vi "PID SP Limiter.vi"(7 "SpLim_State":T2, 8 "REG param":T3={"proportional gain (Kc)"=1.0, "integral time (Ti, s)"=10.0, "derivative time (Td, s)"=1.0, "output high"=100.0, "output high start"=40.0, "output high stop"=40.0, "alr value"=0.0, "output low"=0.0, "output rate (EGU/s)"=5.0, "setpoint max"=100.0, "setpoint rate (EGU/min)"=10.0, "stop rate (EGU/min)"=5.0} {"setpoint max" format="%.2f"; "stop rate (EGU/min)" min=0.001 format="%.2f"; "setpoint rate (EGU/min)" min=0.001 format="%.2f"; "output high stop" format="%.2f"; "output high start" format="%.2f"; "output rate (EGU/s)" min=0.001 format="%.2f"; "output low" format="%.2f"; "alr value" format="%.2f"; "output high" format="%.2f"; "derivative time (Td, s)" format="%.3f"; "integral time (Ti, s)" format="%.3f"; "proportional gain (Kc)" format="%.3f"}, 10 "PV":dbl, 11 "SP":dbl) -> (0 "PID param":T1 {"dt (s)" format="%.3f"; "output rate (EGU/s)" format="%.2f"; "output low" format="%.2f"; "alr value" format="%.2f"; "output high" format="%.2f"; "derivative time (Td, s)" format="%.3f"; "integral time (Ti, s)" format="%.3f"; "proportional gain (Kc)" format="%.3f"}, 1 "End":bool, 2 "T":u32, 3 "output":dbl format="%.2f")   [LabVIEW 2019, in "control.lvlib"]
uses:
  control.lvlib
  ctl/control param.ctl
  ctl/SpLim_State.ctl
  ctl/PID param.ctl
  PID Timing Estimation.vi
panel:
  # "PID gains"
  # "output param"
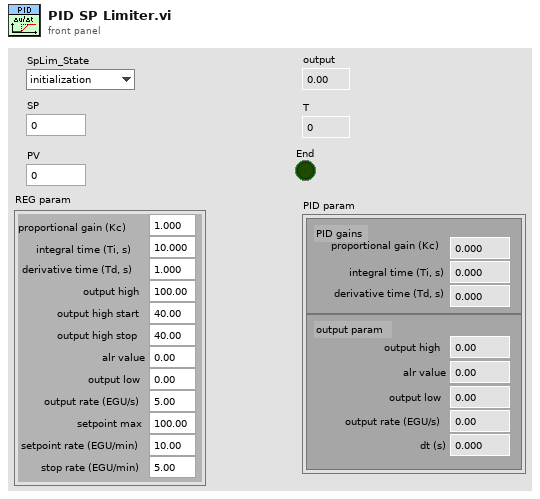
[diagram p1: front panel]
types:
  T1 = typedef "control.lvlib/PID param.ctl" = cluster{"proportional gain (Kc)":dbl, "integral time (Ti, s)":dbl, "derivative time (Td, s)":dbl, "output high":dbl, "alr value":dbl, "output low":dbl, "output rate (EGU/s)":dbl, "dt (s)":dbl}
  T2 = typedef "control.lvlib/SpLim_State.ctl" = enum8{"initialization", "stop", "decrease", "increase"}
  T3 = typedef "control.lvlib/control param.ctl" = cluster{"proportional gain (Kc)":dbl, "integral time (Ti, s)":dbl, "derivative time (Td, s)":dbl, "output high":dbl, "output high start":dbl, "output high stop":dbl, "alr value":dbl, "output low":dbl, "output rate (EGU/s)":dbl, "setpoint max":dbl, "setpoint rate (EGU/min)":dbl, "stop rate (EGU/min)":dbl}
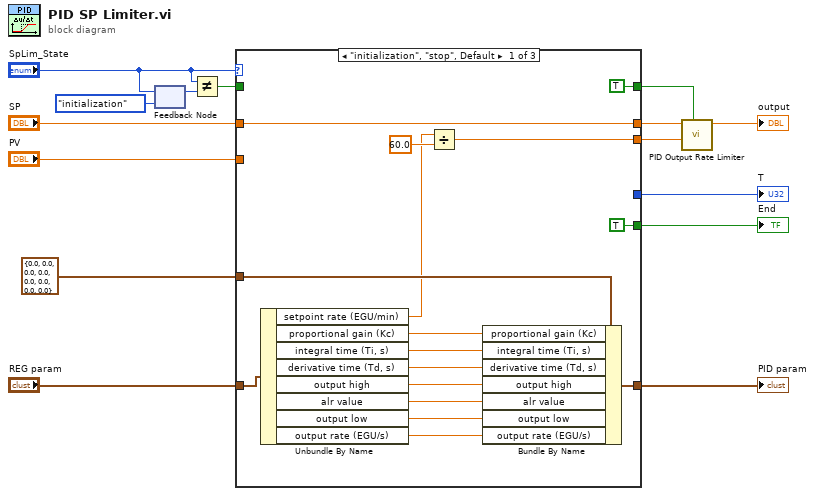
[diagram p0: block diagram]
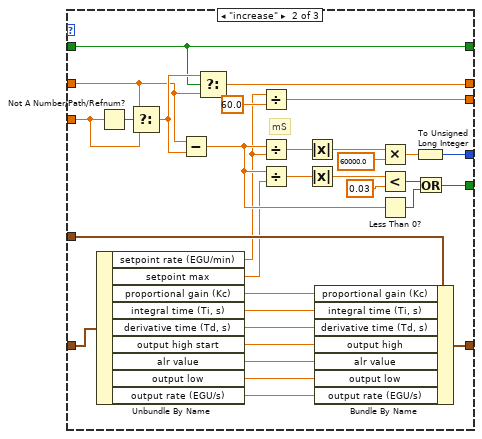
[diagram p2: hidden frame]
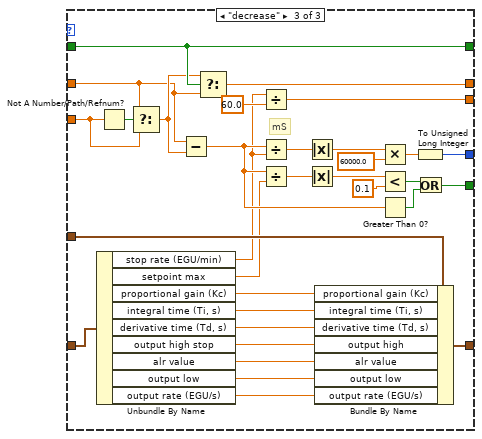
[diagram p3: hidden frame]
diagram:
  n1 = feedback #1(SpLim_State."initialization" ("SpLim_State")) -> (w7:T2)
  n2 = feedback-in #1("SpLim_State") -> ()
  n3 = Not Equal?(x="SpLim_State", y=w7) -> (x != y?=w8:bool)
  n4 = case shown="\"initialization\", \"stop\", Default" "SpLim_State" {
    tunnel: "SP" -> [w31 w37 w67]
    tunnel: "PV" -> [_ w62 w94]
    tunnel: [w31 w34 w71] -> w4
    tunnel: [_ w47 w77] -> w13
    tunnel: [TRUE w43 w75] -> w12
    tunnel: w8 -> [_ w35 w69]
    tunnel: "REG param" -> [w23 w57 w81]
    tunnel: [w22 w49 w80] -> w11
    tunnel: T1 {"proportional gain (Kc)"=0.0, "integral time (Ti, s)"=0.0, "derivative time (Td, s)"=0.0, "output high"=0.0, "alr value"=0.0, "output low"=0.0, "output rate (EGU/s)"=0.0, "dt (s)"=0.0} ("PID param") -> [w21 w38 w73]
    tunnel: [w19 w36 w70] -> w3
    tunnel: [TRUE w35 w69] -> w2
    frame "initialization", "stop", Default {
      n5 = Unbundle By Name(w23) -> ("setpoint rate (EGU/min)"=w18:dbl, "proportional gain (Kc)"=w30:dbl, "integral time (Ti, s)"=w29:dbl, "derivative time (Td, s)"=w28:dbl, "output high"=w27:dbl, "alr value"=w26:dbl, "output low"=w25:dbl, "output rate (EGU/s)"=w24:dbl)
      n6 = Divide(x=w18, y=60.0 ("x")) -> (x/y=w19:dbl)
      n7 = Bundle By Name(cluster=w21, "proportional gain (Kc)"=w30, "integral time (Ti, s)"=w29, "derivative time (Td, s)"=w28, "output high"=w27, "alr value"=w26, "output low"=w25, "output rate (EGU/s)"=w24) -> (w22:T1)
    }
    frame "increase" {
      # "mS"
      n8 = Unbundle By Name(w57) -> ("setpoint rate (EGU/min)"=w33:dbl, "setpoint max"=w32:dbl, "proportional gain (Kc)"=w56:dbl, "integral time (Ti, s)"=w55:dbl, "derivative time (Td, s)"=w54:dbl, "output high start"=w53:dbl, "alr value"=w52:dbl, "output low"=w51:dbl, "output rate (EGU/s)"=w50:dbl)
      n9 = Not A Number/Path/Refnum?(number/path/refnum=w62) -> (NaN/Path/Refnum?=w63:bool)
      n10 = Select(t=w37, s=w63, f=w62) -> (s? t:f=w40:dbl)
      n11 = Subtract(x=w37, y=w40) -> (x-y=w44:dbl)
      n12 = Select(t=w40, s=w35, f=w37) -> (s? t:f=w34:dbl)
      n13 = Divide(x=w33, y=60.0 ("x")) -> (x/y=w36:dbl)
      n14 = Divide(x=w44, y=w33) -> (x/y=w60:dbl)
      n15 = Divide(x=w44, y=w32) -> (x/y=w59:dbl)
      n16 = Absolute Value(x=w60) -> (abs(x)=w46:dbl)
      n17 = Absolute Value(x=w59) -> (abs(x)=w58:dbl)
      n18 = Bundle By Name(cluster=w38, "proportional gain (Kc)"=w56, "integral time (Ti, s)"=w55, "derivative time (Td, s)"=w54, "output high"=w53, "alr value"=w52, "output low"=w51, "output rate (EGU/s)"=w50) -> (w49:T1)
      n19 = Multiply(x=w46, y=60000.0) -> (x*y=w48:dbl)
      n20 = Less?(x=w58, y=0.03) -> (x < y?=w42:bool)
      n21 = Less Than 0?(x=w44) -> (x < 0?=w41:bool)
      n22 = To Unsigned Long Integer(number=w48) -> (unsigned 32bit integer=w47:u32)
      n23 = Or(x=w42, y=w41) -> (x .or. y?=w43:bool)
    }
    frame "decrease" {
      # "mS"
      n24 = Unbundle By Name(w81) -> ("stop rate (EGU/min)"=w65:dbl, "setpoint max"=w64:dbl, "proportional gain (Kc)"=w88:dbl, "integral time (Ti, s)"=w87:dbl, "derivative time (Td, s)"=w86:dbl, "output high stop"=w85:dbl, "alr value"=w84:dbl, "output low"=w83:dbl, "output rate (EGU/s)"=w82:dbl)
      n25 = Not A Number/Path/Refnum?(number/path/refnum=w94) -> (NaN/Path/Refnum?=w95:bool)
      n26 = Select(t=w67, s=w95, f=w94) -> (s? t:f=w68:dbl)
      n27 = Subtract(x=w67, y=w68) -> (x-y=w66:dbl)
      n28 = Select(t=w68, s=w69, f=w67) -> (s? t:f=w71:dbl)
      n29 = Divide(x=w65, y=60.0 ("x")) -> (x/y=w70:dbl)
      n30 = Divide(x=w66, y=w65) -> (x/y=w92:dbl)
      n31 = Divide(x=w66, y=w64) -> (x/y=w91:dbl)
      n32 = Absolute Value(x=w92) -> (abs(x)=w79:dbl)
      n33 = Absolute Value(x=w91) -> (abs(x)=w90:dbl)
      n34 = Bundle By Name(cluster=w73, "proportional gain (Kc)"=w88, "integral time (Ti, s)"=w87, "derivative time (Td, s)"=w86, "output high"=w85, "alr value"=w84, "output low"=w83, "output rate (EGU/s)"=w82) -> (w80:T1)
      n35 = Multiply(x=w79, y=60000.0) -> (x*y=w78:dbl)
      n36 = Less?(x=w90, y=0.1) -> (x < y?=w89:bool)
      n37 = Greater Than 0?(x=w66) -> (x > 0?=w74:bool)
      n38 = To Unsigned Long Integer(number=w78) -> (unsigned 32bit integer=w77:u32)
      n39 = Or(x=w89, y=w74) -> (x .or. y?=w75:bool)
    }
  }
  "PID param" <- w11
  "T" <- w13
  "End" <- w12
  n40 = call "PID Output Rate Limiter.vi"("reinitialize? (F)"=w2, "output rate (EGU/s)"=w3, "input (controller output)"=w4) -> ("output"=→"output":dbl)  [unwired: 7 in, 1 out]
